vi "FindUser.vi"(11 "被查询者的账号":string) -> (3 "Array":string[](array[string]))   [LabVIEW 2020]
uses:
  <vilib>/Utility/file.llb/Read Delimited Spreadsheet (string).vi
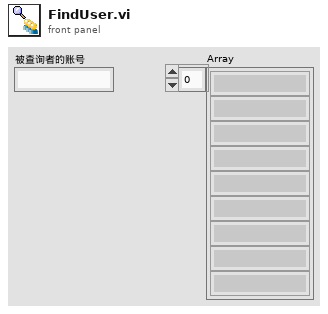
[diagram p1: front panel]
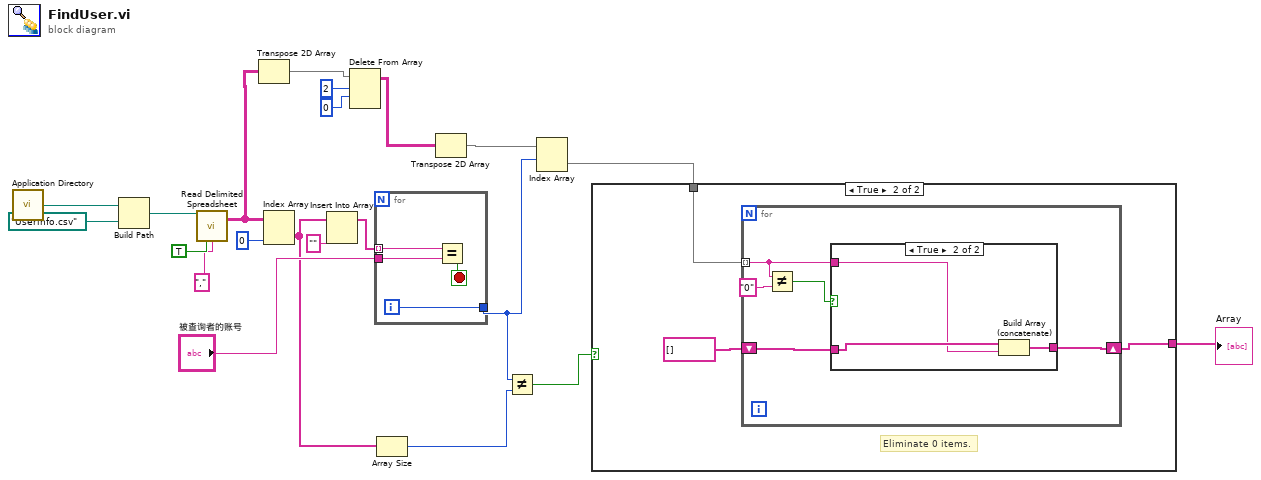
[diagram p0: block diagram]
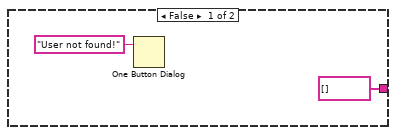
[diagram p2: hidden frame]
diagram:
  n1 = call <vilib>:"Application Directory.vi"() -> ("Application Directory"=w9:path)
  n2 = Build Path(base path=w9, name or relative path=path "Userinfo.csv") -> (appended path=w13:path)
  n3 = call-poly <vilib>:"Read Delimited Spreadsheet.vi"("file path (dialog if empty)"=w13, "transpose? (F)"=TRUE, "delimiter (\\t)"="," ("delimiter (\\t)")) -> ("all rows"=w17:string[][])  [unwired: 7 in, 5 out]
  n4 = Transpose 2D Array(2D array=w17) -> (transposed array=w18:string[][])
  n5 = Index Array(array=w17, index (col)=0 ("index (row)")) -> (element=w1:string[])  [unwired: 1 in]
  n6 = Insert Into Array(array=w1, new element="" ("new element/subarray")) -> (w6:string[])  [unwired: 1 in]
  n7 = Delete From Array(array=w18, length=2, index (row)=0) -> (array with subset deleted=w19:string[][])  [unwired: 1 in, 1 out]
  n8 = for {
    tunnel: w6 -> [w25] mode=indexing
    tunnel: "被查询者的账号" -> [w24]
    tunnel: [w22] -> w5
    i -> [w22]
    stop <- w23 stop-if-true
    n9 = Equal?(x=w25, y=w24) -> (x = y?=w23:bool)
  }
  n10 = Array Size(array=w1) -> (size(s)=w4:i32)
  n11 = Transpose 2D Array(2D array=w19) -> (transposed array=w20:string[][])
  n12 = Not Equal?(x=w5, y=w4) -> (x != y?=w3:bool)
  n13 = Index Array(array=w20, index (row)=w5) -> (element=w21:string[])  [unwired: 1 in]
  n14 = case shown="True" w3 {
    tunnel: w21 -> [_ w30]
    tunnel: [string[] [] w28] -> w2
    frame False {
      n15 = One Button Dialog(message="User not found!") -> ()  [unwired: 1 in, 1 out]
    }
    frame True {
      # "Eliminate 0 items."
      n16 = for {
        shift-right: [w34] -> w28
        shift-left: string[] [] -> [w35]
        tunnel: w30 -> [w32] mode=indexing
        n17 = Not Equal?(x=w32, y="0") -> (x != y?=w31:bool)
        n18 = case shown="True" w31 {
          tunnel: w35 -> [w36 w39]
          tunnel: w32 -> [_ w38]
          tunnel: [w36 w37] -> w34
          frame False {
          }
          frame True {
            n19 = Build Array (concatenate)(w39, w38) -> (w37:string[])
          }
        }
      }
    }
  }
  "Array" <- w2
